vi "GSP_setmenu.vi"(4 "error in (no error)":errorcluster, 6 "GUI States":T1, 7 "menubar":refnum<k9>) -> (0 "error out":errorcluster)   [LabVIEW 2015]
doc: "Sets the main interface menu, to state supplied by GUI States."
uses:
  GUI_states.ctl
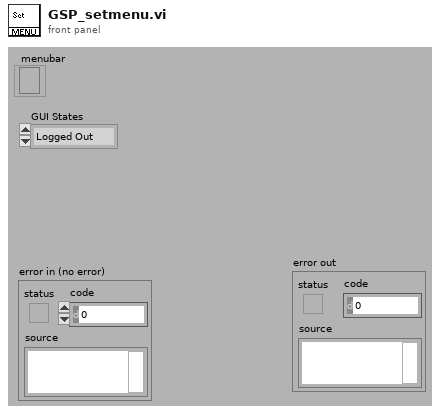
[diagram p1: front panel]
types:
  T1 = typedef "GUI_states.ctl" = enum16{"Logged Out", "Observer", "Operator", "Engineer"}
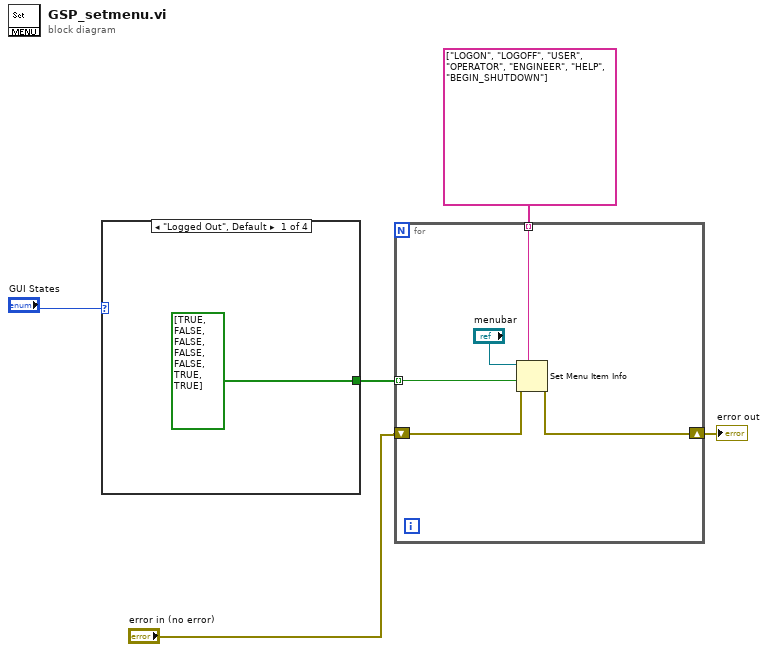
[diagram p0: block diagram]
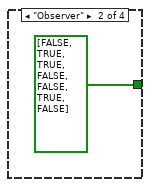
[diagram p2: hidden frame]
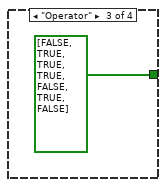
[diagram p3: hidden frame]
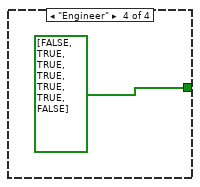
[diagram p4: hidden frame]
diagram:
  n1 = case shown="\"Logged Out\", Default" "GUI States" {
    tunnel: [bool[] [TRUE, FALSE, FALSE, FALSE, FALSE, TRUE, TRUE] bool[] [FALSE, TRUE, TRUE, FALSE, FALSE, TRUE, FALSE] bool[] [FALSE, TRUE, TRUE, TRUE, FALSE, TRUE, FALSE] bool[] [FALSE, TRUE, TRUE, TRUE, TRUE, TRUE, FALSE]] -> w1
    frame "Logged Out", Default {
    }
    frame "Observer" {
    }
    frame "Operator" {
    }
    frame "Engineer" {
    }
  }
  n2 = for {
    shift-right: [w12] -> w3
    shift-left: "error in (no error)" -> [w13]
    tunnel: string[] ["LOGON", "LOGOFF", "USER", "OPERATOR", "ENGINEER", "HELP", "BEGIN_SHUTDOWN"] -> [w11] mode=indexing
    tunnel: w1 -> [w10] mode=indexing
    n3 = Set Menu Item Info(7:w11, 8:w13, 9:w10, 11:"menubar") -> (0:w12:errorcluster)  [unwired: 3 in, 1 out]
  }
  "error out" <- w3
